vi "RT Test.vi"() -> ()   [LabVIEW 2014]
uses:
  Par.ctl
  LambdaType.ctl
  PC_Functions.ctl
  Lambda Ducati Custom Device.lvlib
panel:
  out "counter packets 2":u32
  in  "Cluster 2":T1={"local port"=5559, "receiver address"=0, "connection ID"=refnum, "receiver port"=5559}
  in  "Array 4":dbl[](array[numeric])=[1.0, 0.0, 2.0, 0.01, 0.0, 0.1, 1000.0, 0.0, 0.0, 0.0, 2.0, 0.01, 0.0, 0.1, 1000.0, 0.0, 0.0]
  out "Array 3":dbl[](array[numeric]) format="%#_3g"
  in  "Count(mSec) 2":u32=5
  out "dt 2":u32
  in  "par 3":T2={"Loop time"={"Period [ms]"=0, "Processor"=0}, "COM"={"COM IP"="192.168.8.71", "COM port"=30006, "Local port"=5557}, "Lambda Type"=enum."LSU4.2", "Lambda"={"LSU4.2 Lambda"=[], "LSU4.2 Ip"=[], "LSU4.9 Lambda"=[], "LSU4.9 Ip"=[], "LZA03 Lambda"=[], "LZA03 Ip"=[], "NTK Lambda"=[], "NTK Ip"=[], "Custom Lambda"=[], "Custom Ip"=[]}, "Ro_0 [Ohm]"=0.0, "Ro_1 [Ohm]"=0.0}
  in  "error in 2":errorcluster
  out "error out 2":errorcluster
  out "dt":u32
  out "counter packets":u32
  in  "Count(mSec)":u32=5
  out "error out":errorcluster
  in  "error in":errorcluster
  out "Array out":dbl[](array[numeric]) format="%#_3g"
  in  "Array":dbl[](array[numeric])=[1.0, 0.0, 2.0, 0.01, 0.0, 0.1, 1000.0, 0.0, 0.0, 0.0, 2.0, 0.01, 0.0, 0.1, 1000.0, 0.0, 0.0]
  in  "par 2":T2={"Loop time"={"Period [ms]"=0, "Processor"=0}, "COM"={"COM IP"="192.168.8.70", "COM port"=30005, "Local port"=5556}, "Lambda Type"=enum."LSU4.2", "Lambda"={"LSU4.2 Lambda"=[], "LSU4.2 Ip"=[], "LSU4.9 Lambda"=[], "LSU4.9 Ip"=[], "LZA03 Lambda"=[], "LZA03 Ip"=[], "NTK Lambda"=[], "NTK Ip"=[], "Custom Lambda"=[], "Custom Ip"=[]}, "Ro_0 [Ohm]"=0.0, "Ro_1 [Ohm]"=0.0}
  in  "Cluster":T1={"local port"=5559, "receiver address"=0, "connection ID"=refnum, "receiver port"=5559}
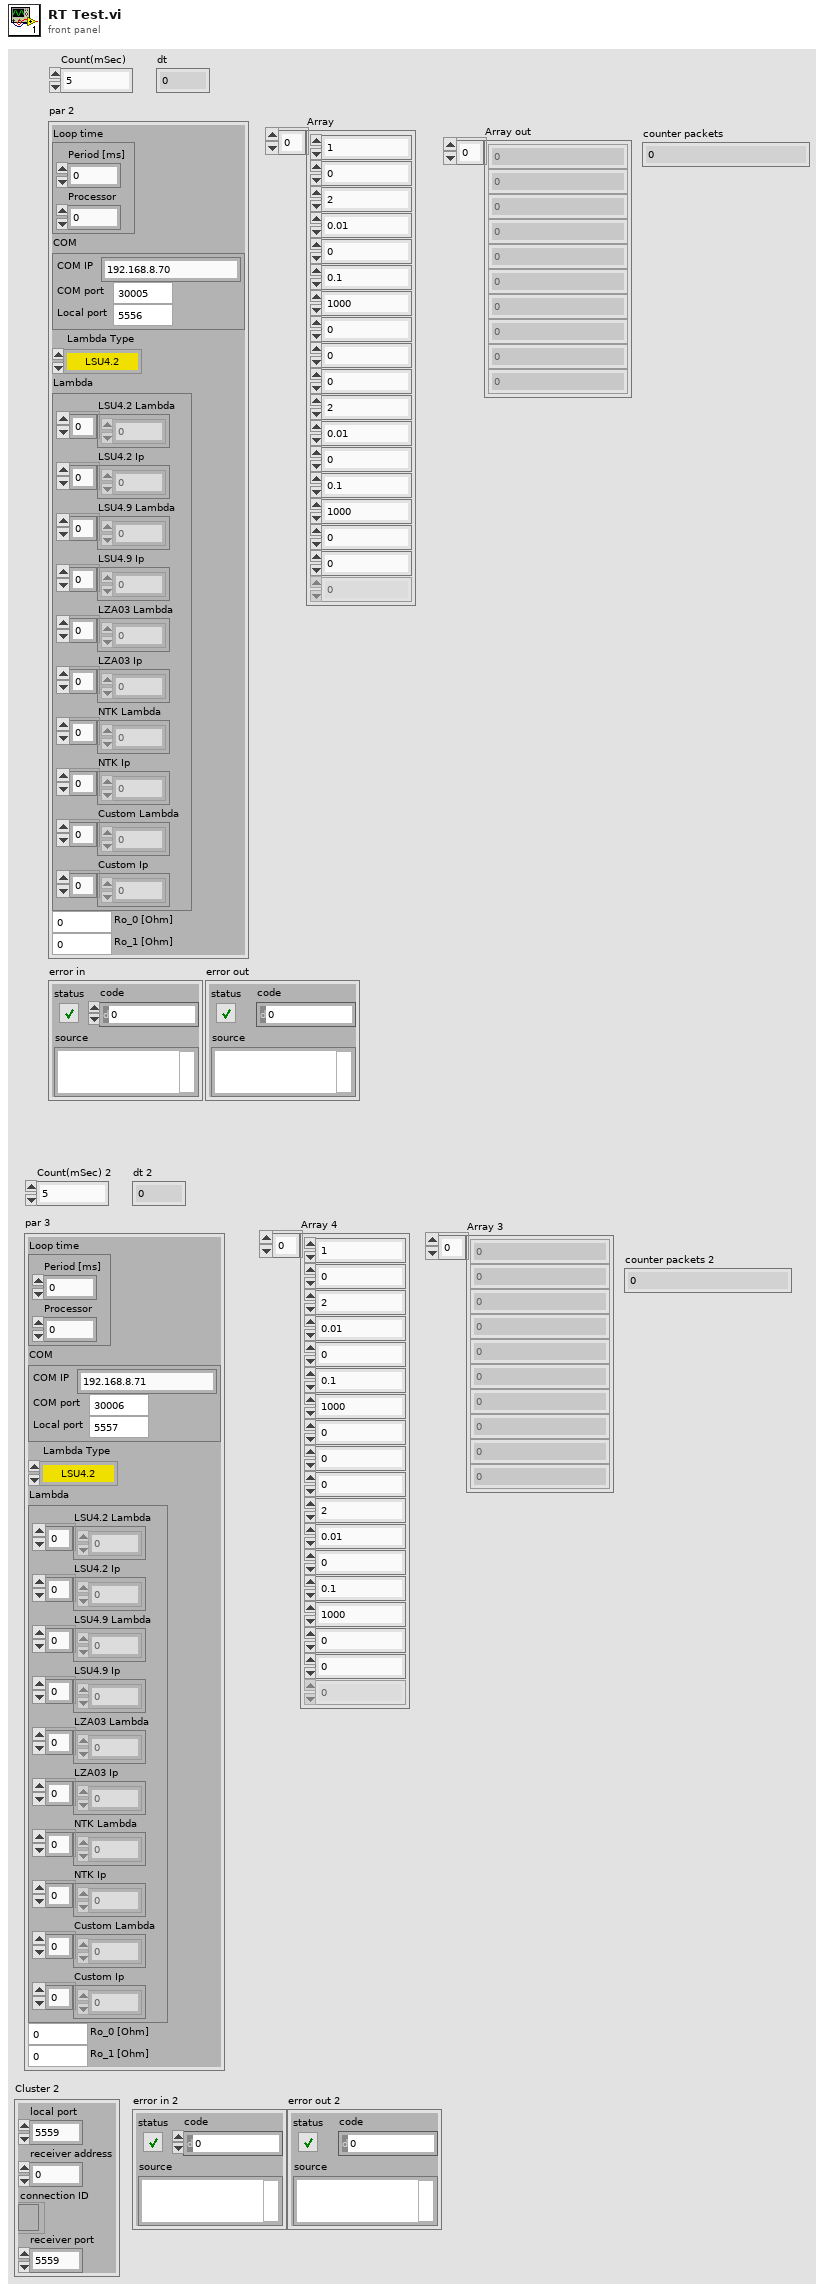
[diagram p1: front panel]
types:
  T1 = cluster{"local port":u16, "receiver address":u32, "connection ID":refnum<k16>, "receiver port":u16}
  T2 = typedef "Lambda Ducati Custom Device.lvlib/Par.ctl" = cluster{"Loop time":cluster{"Period [ms]":i64, "Processor":i32}, "COM":cluster{"COM IP":string, "COM port":u64, "Local port":u64}, "Lambda Type":T3, "Lambda":cluster{"LSU4.2 Lambda":dbl[], "LSU4.2 Ip":dbl[], "LSU4.9 Lambda":dbl[], "LSU4.9 Ip":dbl[], "LZA03 Lambda":dbl[], "LZA03 Ip":dbl[], "NTK Lambda":dbl[], "NTK Ip":dbl[], "Custom Lambda":dbl[], "Custom Ip":dbl[]}, "Ro_0 [Ohm]":dbl, "Ro_1 [Ohm]":dbl}
  T3 = typedef "LambdaType.ctl" = enum16{"LSU4.2", "Bosch", "LZA03", "LZA08", "Custom", "[mA]"}
  T4 = typedef "Lambda Ducati Custom Device.lvlib/PC_Functions.ctl" = enum16{"Initialize", "Send", "Idle", "Exit"}
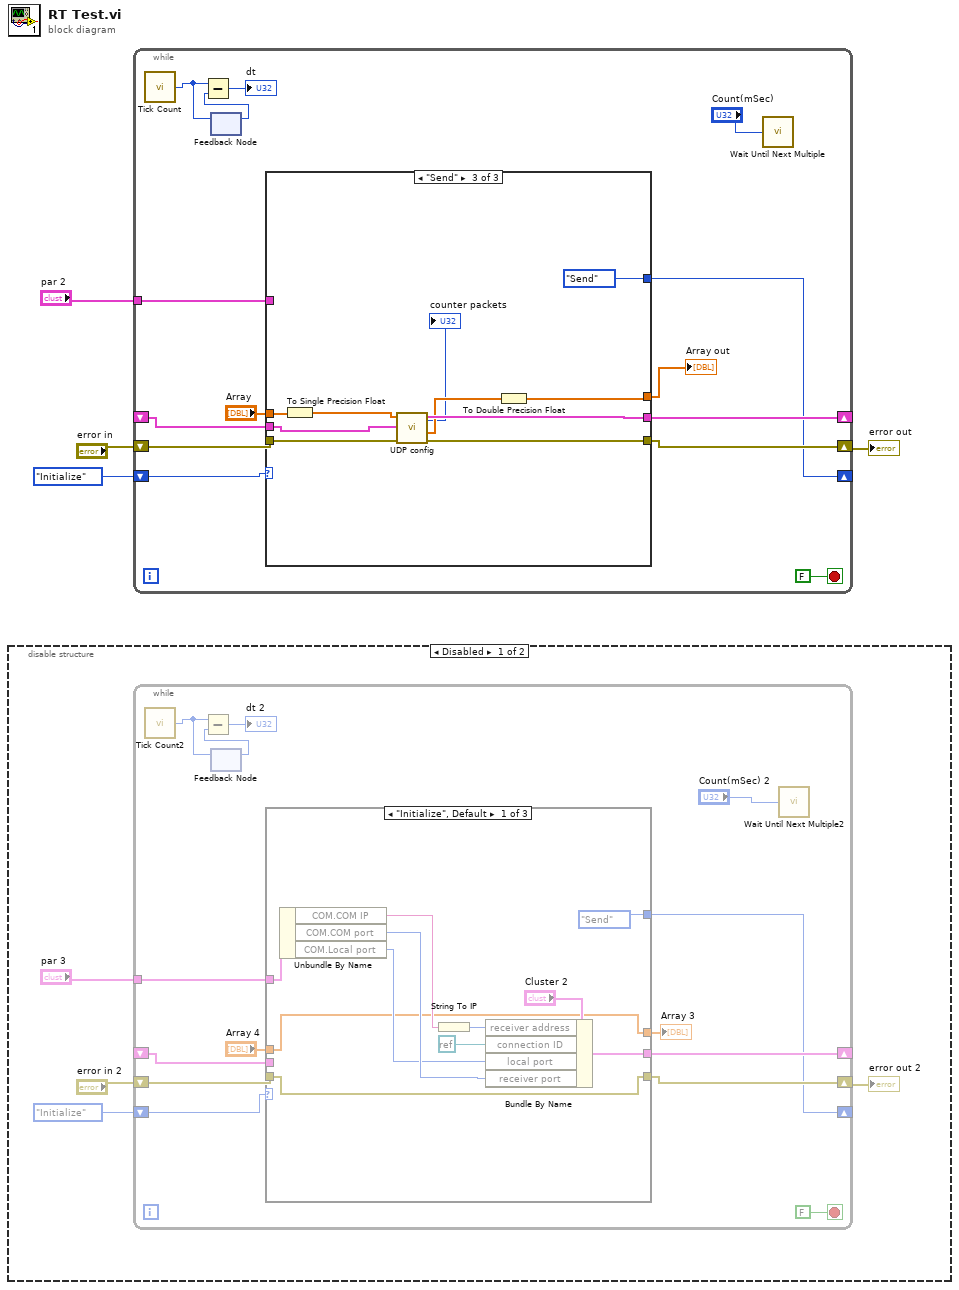
[diagram p0: block diagram]
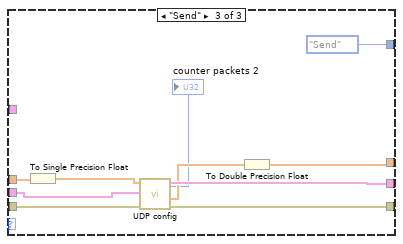
[diagram p3: hidden frame]
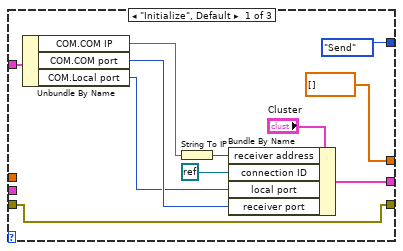
[diagram p5: hidden frame]
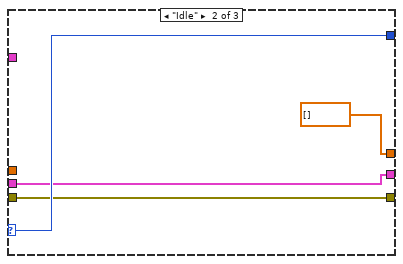
[diagram p6: hidden frame]
diagram:
  n1 = disable-structure shown="Disabled" {
    frame Disabled {
      n2 = while {
        tunnel: "par 3" -> [w20]
        shift-right: [w16] -> w7
        shift-left: "error in 2" -> [w17]
        shift-right: [w15] -> _
        shift-left: _ -> [w14]
        shift-right: [w12] -> _
        shift-left: PC_Functions."Initialize" ("Command") -> [w13]
        stop <- FALSE stop-if-true
        n3 = call "Tick Count2"() -> ("Tick Count(mSec)"=w11:u32)
        n4 = feedback-in #1(w11) -> ()
        n5 = feedback #1() -> (w10:u32)  [unwired: 1 in]
        n6 = Subtract(x=w11, y=w10) -> (x-y=→"dt 2":u32)
        n7 = case shown="\"Initialize\", Default" w13 {
          selector: w13 -> [_ w37 _]
          tunnel: [w30 w34 w46] -> w15
          tunnel: w17 -> [w24 w36 w44]
          tunnel: [w24 w36 w45] -> w16
          tunnel: [PC_Functions."Send" ("Command") w37 PC_Functions."Send" ("Command")] -> w12
          tunnel: "Array 4" -> [w23 w35 w43]
          tunnel: [w23 w35 w42] -> w18
          tunnel: w20 -> [w28 _ _]
          tunnel: w14 -> [_ w34 w41]
          frame "Initialize", Default {
            n8 = Unbundle By Name(w28) -> ("COM.COM IP"=w27:string, "COM.COM port"=w26:u64, "COM.Local port"=w25:u64)
            n9 = String To IP(1:w27) -> (0:w32:u32)
            n10 = Bundle By Name(cluster="Cluster 2", "receiver address"=w32, "connection ID"=refnum<k0> refnum, "local port"=w25, "receiver port"=w26) -> (w30:T1)
          }
          frame "Idle" {
          }
          frame "Send" {
            n11 = To Single Precision Float(number=w43) -> (single precision float=w40:sgl[])
            n12 = call "UDP config.vi"("error in"=w44, "Cluster in"=w41, "Data In"=w40) -> ("error out"=w45:errorcluster, "Data Out"=w39:sgl[], "Cluster out"=w46:T1, "counter packets"=→"counter packets 2":u32)  [unwired: 4 in, 1 out]
            n13 = To Double Precision Float(number=w39) -> (double precision float=w42:dbl[])
          }
        }
        "Array 3" <- w18
        n14 = call "Wait Until Next Multiple2"("Count(mSec)"="Count(mSec) 2") -> ()  [unwired: 1 out]
      }
      "error out 2" <- w7
    }
    frame Enabled {
    }
  }
  n15 = while {
    tunnel: "par 2" -> [w59]
    shift-right: [w56] -> w2
    shift-left: "error in" -> [w57]
    shift-right: [w55] -> _
    shift-left: _ -> [w54]
    shift-right: [w52] -> _
    shift-left: PC_Functions."Initialize" ("Command") -> [w53]
    stop <- FALSE stop-if-true
    n16 = call "Tick Count"() -> ("Tick Count(mSec)"=w51:u32)
    n17 = feedback-in #2(w51) -> ()
    n18 = feedback #2() -> (w50:u32)  [unwired: 1 in]
    n19 = Subtract(x=w51, y=w50) -> (x-y=→"dt":u32)
    n20 = case shown="\"Send\"" w53 {
      selector: w53 -> [_ w76 _]
      tunnel: [w69 w74 w85] -> w55
      tunnel: w57 -> [w63 w75 w83]
      tunnel: [w63 w75 w84] -> w56
      tunnel: [PC_Functions."Send" ("Command") w76 PC_Functions."Send" ("Command")] -> w52
      tunnel: "Array" -> [_ _ w82]
      tunnel: [dbl[] [] ("Array") dbl[] [] ("Array") w81] -> w48
      tunnel: w59 -> [w67 _ _]
      tunnel: w54 -> [_ w74 w80]
      frame "Initialize", Default {
        n21 = Unbundle By Name(w67) -> ("COM.COM IP"=w66:string, "COM.COM port"=w65:u64, "COM.Local port"=w64:u64)
        n22 = String To IP(1:w66) -> (0:w71:u32)
        n23 = Bundle By Name(cluster="Cluster", "receiver address"=w71, "connection ID"=refnum<k0> refnum, "local port"=w64, "receiver port"=w65) -> (w69:T1)
      }
      frame "Idle" {
      }
      frame "Send" {
        n24 = To Single Precision Float(number=w82) -> (single precision float=w79:sgl[])
        n25 = call "UDP config.vi"("error in"=w83, "Cluster in"=w80, "Data In"=w79) -> ("error out"=w84:errorcluster, "Data Out"=w78:sgl[], "Cluster out"=w85:T1, "counter packets"=→"counter packets":u32)  [unwired: 4 in, 1 out]
        n26 = To Double Precision Float(number=w78) -> (double precision float=w81:dbl[])
      }
    }
    "Array out" <- w48
    n27 = call "Wait Until Next Multiple"("Count(mSec)"="Count(mSec)") -> ()  [unwired: 1 out]
  }
  "error out" <- w2
